vi "DAQ 모터 다루기 실습(카운터, 디지털 입력).vi"() -> ()   [LabVIEW 2020]
uses:
  <vilib>/DAQmx/read.llb/DAQmx Read (Digital 1D Bool 1Chan 1Samp).vi
  <vilib>/DAQmx/create/channels.llb/DAQmx Create Channel (CO-Pulse Generation-Frequency).vi
  <vilib>/DAQmx/configure/timing.llb/DAQmx Timing (Implicit).vi
  <vilib>/DAQmx/create/channels.llb/DAQmx Create Channel (DI-Digital Input).vi
  <vilib>/DAQmx/miscellaneous.llb/DAQmx Fill In Error Info.vi
panel:
  out "출력 클러스터":cluster{i16, i16, i16}(graph)
  out "data":bool[](array[boolean]) caption="데이터"
  in  "정지":bool
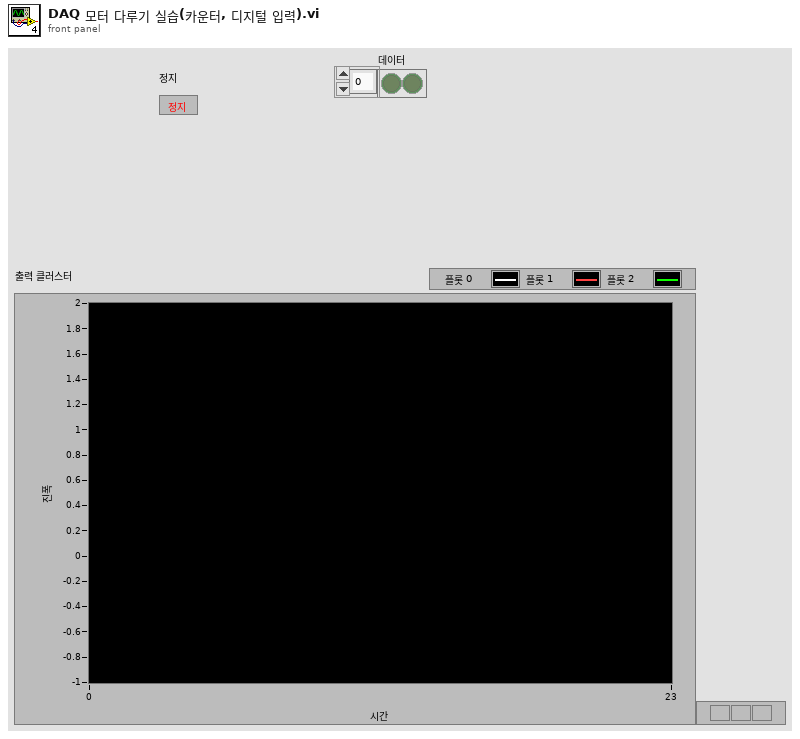
[diagram p1: front panel]
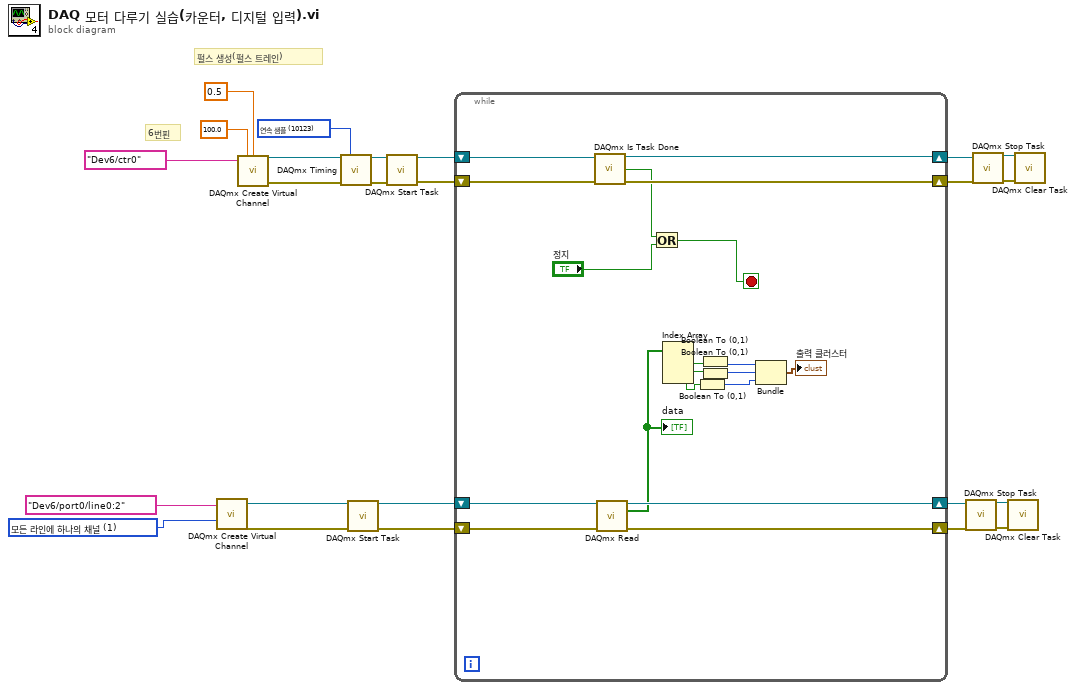
[diagram p0: block diagram]
diagram:
  w9 = 1 items=["각 라인에 하나의 채널", "모든 라인에 하나의 채널"] ("line grouping")
  w21 = 10123 items=["유한 샘플"=10178, "연속 샘플"=10123, "하드웨어 타이밍에 의한 단일 포인트"=12522] ("sample mode")
  # "펄스 생성(펄스 트레인)"
  # "6번핀"
  n1 = call-poly <vilib>:"DAQmx Create Virtual Channel.vi"("lines"=tag "Dev6/port0/line0:2", "line grouping"=w9) -> ("task out"=w8:refnum<k21>, "error out"=w7:errorcluster)  [unwired: 12 in]
  n2 = call-poly <vilib>:"DAQmx Create Virtual Channel.vi"("frequency"=100.0, "duty cycle"=0.5, "counter"=tag "Dev6/ctr0") -> ("task out"=w23:refnum<k21>, "error out"=w22:errorcluster)  [unwired: 11 in]
  n3 = call-poly <vilib>:"DAQmx Timing.vi"("task/channels in"=w23, "sample mode"=w21, "error in"=w22) -> ("task out"=w18:refnum<k21>, "error out"=w17:errorcluster)  [unwired: 11 in]
  n4 = call <vilib>:"DAQmx Start Task.vi"("task/channels in"=w8, "error in"=w7) -> ("task out"=w6:refnum<k21>, "error out"=w5:errorcluster)  [unwired: 12 in]
  n5 = call <vilib>:"DAQmx Start Task.vi"("task/channels in"=w18, "error in"=w17) -> ("task out"=w16:refnum<k21>, "error out"=w15:errorcluster)  [unwired: 12 in]
  n6 = while {
    shift-right: [w41] -> w14
    shift-left: w16 -> [w43]
    shift-right: [w40] -> w13
    shift-left: w15 -> [w42]
    shift-right: [w34] -> w2
    shift-left: w6 -> [w36]
    shift-right: [w33] -> w1
    shift-left: w5 -> [w35]
    stop <- w37 stop-if-true
    n7 = call <vilib>:"DAQmx Is Task Done.vi"("task/channels in"=w43, "error in"=w42) -> ("task out"=w41:refnum<k21>, "task done?"=w39:bool, "error out"=w40:errorcluster)  [unwired: 11 in]
    n8 = call-poly <vilib>:"DAQmx Read.vi"("task/channels in"=w36, "error in"=w35) -> ("task out"=w34:refnum<k21>, "data"=w32:bool[], "error out"=w33:errorcluster)  [unwired: 11 in]
    "data" <- w32
    n9 = Or(x=w39, y="정지") -> (x .or. y?=w37:bool)
    n10 = Index Array(array=w32) -> (element #1=w31:bool, element #2=w30:bool, element #3=w27:bool)  [unwired: 3 in]
    n11 = Boolean To (0,1)(Boolean=w27) -> (0, 1=w26:i16)
    n12 = Boolean To (0,1)(Boolean=w31) -> (0, 1=w29:i16)
    n13 = Boolean To (0,1)(Boolean=w30) -> (0, 1=w28:i16)
    n14 = Bundle(w29, w28, w26) -> (→"출력 클러스터":cluster{i16, i16, i16})  [unwired: 1 in]
  }
  n15 = call <vilib>:"DAQmx Stop Task.vi"("task/channels in"=w2, "error in"=w1) -> ("task out"=w3:refnum<k21>, "error out"=w4:errorcluster)  [unwired: 12 in]
  n16 = call <vilib>:"DAQmx Stop Task.vi"("task/channels in"=w14, "error in"=w13) -> ("task out"=w12:refnum<k21>, "error out"=w11:errorcluster)  [unwired: 12 in]
  n17 = call <vilib>:"DAQmx Clear Task.vi"("task in"=w3, "error in"=w4) -> ()  [unwired: 13 in, 1 out]
  n18 = call <vilib>:"DAQmx Clear Task.vi"("task in"=w12, "error in"=w11) -> ()  [unwired: 13 in, 1 out]
